vi "8bit sync-Resize cam video.vi"(4 "Funct exporter":bool, 6 "Initial frame":bool, 7 "Required cam video height":u32=94, 8 "error in (no error)":errorcluster, 9 "Frame number (unity based)":i32, 10 "Ctrl refs":T2, 11 "Microscope image":T1) -> (0 "error out":errorcluster, 2 "Resampled Cam video":T1, 3 "X Resolution of speed graph":u32)   [LabVIEW 2020]
uses:
  Timelapse Viewer/Typedefs/8-bit video export window ctrl refs.ctl
  Typedefs/Bright-Contr-Gamma cluster.ctl
  Timelapse Viewer/Typedefs/Speed graph behaviour enum.ctl
  <vilib>/vision/Image Controls.llb/IMAQ Image.ctl
  Functional Imaging Viewer/Typedefs/Get-Set-Clear Control.ctl
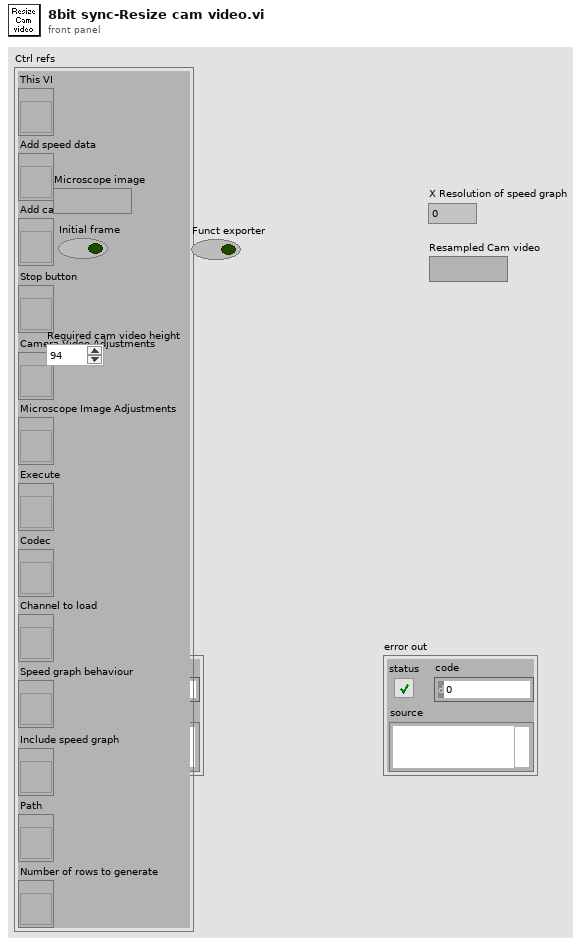
[diagram p1: front panel]
types:
  T1 = typedef "IMAQ Image.ctl" = refnum<image>
  T2 = typedef "8-bit video export window ctrl refs.ctl" = cluster{"This VI":refnum<vi>, "Add speed data":refnum<vi>, "Add camera videos":refnum<vi>, "Stop button":refnum<vi>, "Camera Video Adjustments":refnum<vi>, "Microscope Image Adjustments":refnum<vi>, "Execute":refnum<vi>, "Codec":refnum<vi>, "Channel to load":refnum<vi>, "Speed graph behaviour":refnum<vi>, "Include speed graph":refnum<vi>, "Number of rows to generate":refnum<vi>, "Path":refnum<vi>}
  T3 = typedef "Get-Set-Clear Control.ctl" = enum16{"Get", "Set", "Clear"}
  T4 = typedef "Cam videos cluster.ctl" = cluster{"Vid 1":T1, "Vid 2":T1, "Vid 3":T1, "Vid 4":T1, "Vid1 Rel time (ms)":u32, "Vid2 Rel time (ms)":u32, "Vid3 Rel time (ms)":u32, "Vid4 Rel time (ms)":u32}
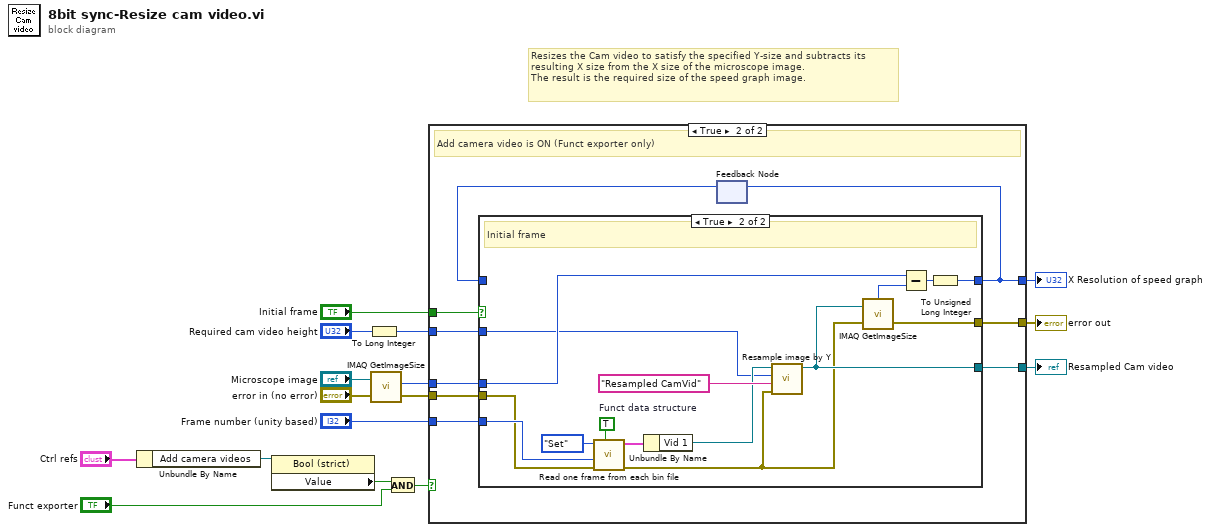
[diagram p0: block diagram]
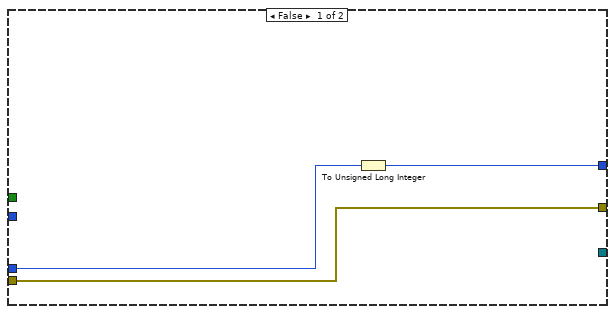
[diagram p2: hidden frame]
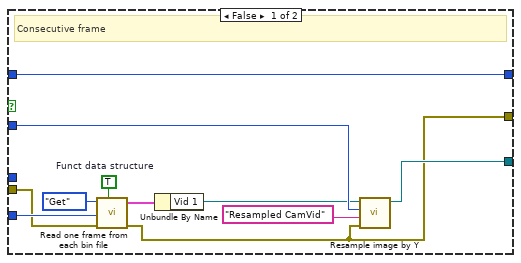
[diagram p3: hidden frame]
diagram:
  # "Resizes the Cam video to satisfy the specified Y-size and subtracts its resulting X size from the X size of the microscope image.\nThe result is the required size of the speed graph image."
  n1 = Unbundle By Name("Ctrl refs") -> ("Add camera videos"=w6:refnum<vi>)
  n2 = property class="Bool (strict)"(reference=w6) -> ("Value"=w7:bool)  [unwired: 1 in, 2 out]
  n3 = To Long Integer(number="Required cam video height") -> (32bit integer=w4:i32)
  n4 = call "IMAQ GetImageSize"("Image"="Microscope image", "error in (no error)"="error in (no error)") -> ("X Resolution"=w10:i32, "error out"=w8:errorcluster)  [unwired: 3 out]
  n5 = And(x=w7, y="Funct exporter") -> (x .and. y?=w1:bool)
  n6 = case shown="True" w1 {
    tunnel: [w18 w28] -> w16
    tunnel: [_ w27] -> w15
    tunnel: "Initial frame" -> [_ w26]
    tunnel: [w17 w25] -> w13
    tunnel: "Frame number (unity based)" -> [_ w23]
    tunnel: w10 -> [w19 w22]
    tunnel: w8 -> [w18 w21]
    tunnel: w4 -> [_ w20]
    frame False {
      n7 = To Unsigned Long Integer(number=w19) -> (unsigned 32bit integer=w17:u32)
    }
    frame True {
      # "Add camera video is ON (Funct exporter only)"
      n8 = feedback #1() -> (w24:u32)  [unwired: 1 in]
      n9 = case shown="True" w26 {
        tunnel: w21 -> [w32 w41]
        tunnel: [w31 w54] -> w28
        tunnel: [w33 w53] -> w27
        tunnel: [w39 w52] -> w25
        tunnel: w24 -> [w39 _]
        tunnel: w20 -> [w30 w40]
        tunnel: w23 -> [w34 w50]
        tunnel: w22 -> [_ w49]
        frame False {
          w36 = TRUE  # Funct data structure
          # "Consecutive frame"
          n10 = call "Read one frame from each bin file.vi"("Funct data structure"=w36, "error in (no error)"=w32, "Master video's frame number (unity-based)"=w34, "Get/set"=Get-Set-Clear_Control."Get" ("GEt set .bin refs")) -> ("Error out"=w31:errorcluster, "Cam videos cluster"=w35:T4)  [unwired: 6 in]
          n11 = Unbundle By Name(w35) -> ("Vid 1"=w29:T1)
          n12 = call "Resample image by Y.vi"("error in (no error)"=w31, "Resampled Image Name"="Resampled CamVid", "Y Resolution"=w30, "Refnum in"=w29) -> ("Refnum out"=w33:T1)  [unwired: 7 in]
        }
        frame True {
          w46 = TRUE  # Funct data structure
          # "Initial frame"
          n13 = call "Read one frame from each bin file.vi"("Funct data structure"=w46, "error in (no error)"=w41, "Master video's frame number (unity-based)"=w50, "Get/set"=Get-Set-Clear_Control."Set" ("GEt set .bin refs")) -> ("Error out"=w42:errorcluster, "Cam videos cluster"=w45:T4)  [unwired: 6 in]
          n14 = Unbundle By Name(w45) -> ("Vid 1"=w44:T1)
          n15 = call "Resample image by Y.vi"("error in (no error)"=w42, "Resampled Image Name"="Resampled CamVid", "Y Resolution"=w40, "Refnum in"=w44) -> ("Refnum out"=w53:T1)  [unwired: 7 in]
          n16 = call "IMAQ GetImageSize"("Image"=w53, "error in (no error)"=w42) -> ("X Resolution"=w43:i32, "error out"=w54:errorcluster)  [unwired: 3 out]
          n17 = Subtract(x=w49, y=w43) -> (x-y=w51:i32)
          n18 = To Unsigned Long Integer(number=w51) -> (unsigned 32bit integer=w52:u32)
        }
      }
      n19 = feedback-in #1(w25) -> ()
    }
  }
  "error out" <- w16
  "X Resolution of speed graph" <- w13
  "Resampled Cam video" <- w15
